vi "Service ID.vi"(8 "error in (no error)":errorcluster, 11 "Password Encoder in":refnum<class "Password Encoder.lvclass">) -> (0 "error out":errorcluster, 2 "Service ID":string, 3 "Password Encoder out":refnum<class "Password Encoder.lvclass">)   [LabVIEW 2020, in "HTTP Server.lvlib" / "Password Encoder.lvclass"]
uses:
  Password Encoder.lvclass
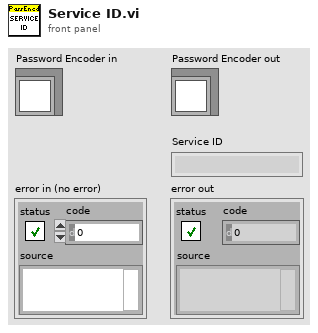
[diagram p1: front panel]
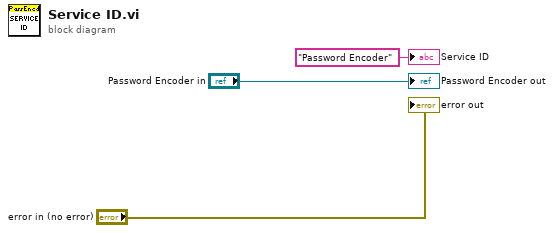
[diagram p0: block diagram]
diagram:
  "error out" <- "error in (no error)"
  "Password Encoder out" <- "Password Encoder in"
  "Service ID" <- "Password Encoder" ("Service ID")
